vi "2_AdvancedDemo_HHHisto.vi"() -> ()   [LabVIEW 2010]
uses:
  Types/HH_UIThread_Cmds.ctl
  _lib/PQ/HydraHarp/HH_InitInfo.ctl
  Types/HH_UIThread_Data.ctl
  Types/HH_InputChannel.ctl
  _lib/PQ/HydraHarp/HH_RefSource.ctl
  _lib/PQ/HydraHarp/HH_MeasMode.ctl
  _lib/PQ/HydraHarp/hhlib_x86_x64_UIThread.llb/HH_DllPath_global.vi
  <vilib>/Utility/error.llb/DialogType.ctl
  _lib/PQ/HydraHarp/HH_LibVersion_global.vi
panel:
  in  "Settings":bool=TRUE
  in  "Run continuously":bool=TRUE caption="Conti."
  in  "Start":bool
  in  "Scale":bool
  out "CountRates":i32[](graph)
  in  "HistoLength":i32(ring)=6 caption="Num Bins" items=["1024", "2048", "4096", "8192", "16384", "32768", "65536"]
  in  "OvlLevel":u32=4294967295 caption="Ovl.Level" min=1 step=1
  in  "StopOvl.":bool=TRUE
  in  "AcqTime":i32=1000 caption="Acqu.     ms" min=1 max=360000000 step=1
  in  "Binning":i32(ring) caption="Resol.      ps" items=["1", "2", "4", "8", "16", "32", "64", "128", "256", "512", "1024", "2048", "4096", "8192", "16384", "32768", "65536", "131072", "262144", "524288", "1048576", "2097152", "4194304", "8388608", "16777216", "33554432"]
  in  "HistoOffset":i32 caption="Offset      ns" min=0 max=500000 step=1
  out "HistoGraph":T1(graph)={0.0, "Resolution"=0.001, "Histogram"=array8x1024[8192 elements]}
  in  "SyncZeroX":i32=10 caption="ZeroCr.  mV" min=0 max=40 step=1
  in  "SyncDivider":i32(ring)=3 caption="Divider" items=["1", "2", "4", "8", "16"]
  in  "SyncOffset":i32 caption="Offset      ps" min=-99999 max=99999 step=1
  in  "SyncLevel":i32=50 caption="Level      mV" min=0 max=1000 step=1
  in  "Channels":T2[](array[typedef])=[{"Name"="Inp.Chan 1", "Enable"=TRUE, "Offset"=0, "CFDLevel"=50, "ZeroX"=10}, {"Name"="Inp.Chan 2", "Enable"=TRUE, "Offset"=0, "CFDLevel"=50, "ZeroX"=10}, {"Name"="Inp.Chan 3", "Enable"=TRUE, "Offset"=0, "CFDLevel"=50, "ZeroX"=10}, {"Name"="Inp.Chan 4", "Enable"=TRUE, "Offset"=0, "CFDLevel"=50, "ZeroX"=10}, {"Name"="Inp.Chan 5", "Enable"=TRUE, "Offset"=0, "CFDLevel"=50, "ZeroX"=10}, {"Name"="Inp.Chan 6", "Enable"=TRUE, "Offset"=0, "CFDLevel"=50, "ZeroX"=10}, {"Name"="Inp.Chan 7", "Enable"=TRUE, "Offset"=0, "CFDLevel"=50, "ZeroX"=10}, {"Name"="Inp.Chan 8", "Enable"=TRUE, "Offset"=0, "CFDLevel"=50, "ZeroX"=10}] {"ZeroX" min=0 max=40 step=1; "Offset" min=-99999 max=99999 step=1; "CFDLevel" min=0 max=1000 step=1}
  out "SyncRate":string="Sync Rate: 0 cps\n"
  out "OverFlow":bool caption="Overflow:"
  out "Status":string="Initialized!"
  # "Histogram"
  # "Sync"
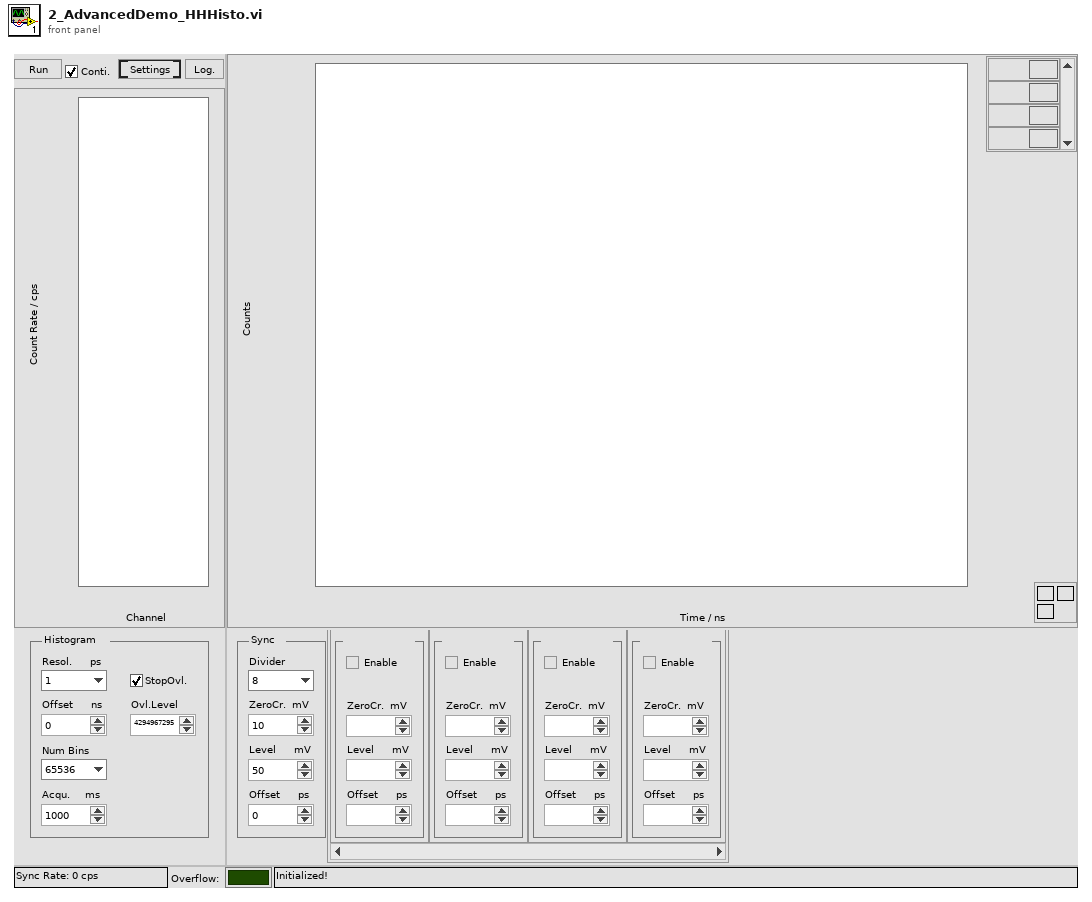
[diagram p1: front panel]
types:
  T1 = cluster{dbl, "Resolution":dbl, "Histogram":u32[][]}
  T2 = typedef "HH_InputChannel.ctl" = cluster{"Name":string, "Enable":bool, "Offset":i32, "CFDLevel":i32, "ZeroX":i32}
  T3 = typedef "HH_UIThread_Data.ctl" = cluster{"Init Info":T4, "DevIdx":i32, "SyncDivider":i32, "SyncOffset":i32, "SyncLevel":i32, "Channels":T2[], "CurrentChannels":i32[], "AcqTime":i32, "Binning":i32, "HistoOffset":i32, "HistoLen":i32, "StopOvl.":bool, "OvlLevel":u32, "StartMeas":bool, "HistoLength":i32, "Resolution":dbl, "Run cont.":bool, "Status":string, "SyncRate":i32, "BitShift":i32, "HistoAcqTime":dbl, "SyncZeroX":i32, "SyncRateStart":i32}
  T4 = typedef "HH_InitInfo.ctl" = cluster{"Library Version":string, "Serial No.":string, "Model":string, "Partnum":string, "Version":string, "features":i32, "nchannels":i32, "nummod":i32, "Model Codes":i32[], "Version Codes":i32[], "Base Resolution":dbl, "Bin Steps":i32}
  T5 = typedef "HH_UIThread_Cmds.ctl" = enum16{"Idle", "Init", "SetInpChanEnable", "SetInpChanOffset", "SetInpChanTrg", "SetSyncDivider", "SetSyncTrg", "SetSyncOffset", "SetBinning", "SetHistoOffset", "SetHistoLen", "SetStopOvl", "SetBitShift", "SetHistoAcqTime", "GetRates", "StartMeas", "StopMeas", "AbortMeas", "GetResolution", "GetHisto", "ReadFiFo", "WriteStatus", "Resize", "EnableControls", "DisableControls", "Error", "Exit"}
  T6 = enum8{"Enabled", "Disabled", "Disabled and Grayed Out"}
  T7 = typedef "HH_MeasMode.ctl" = i32
  T8 = typedef "HH_RefSource.ctl" = enum16{"internal", "external"}
  T9 = typedef "DialogType.ctl" = u16
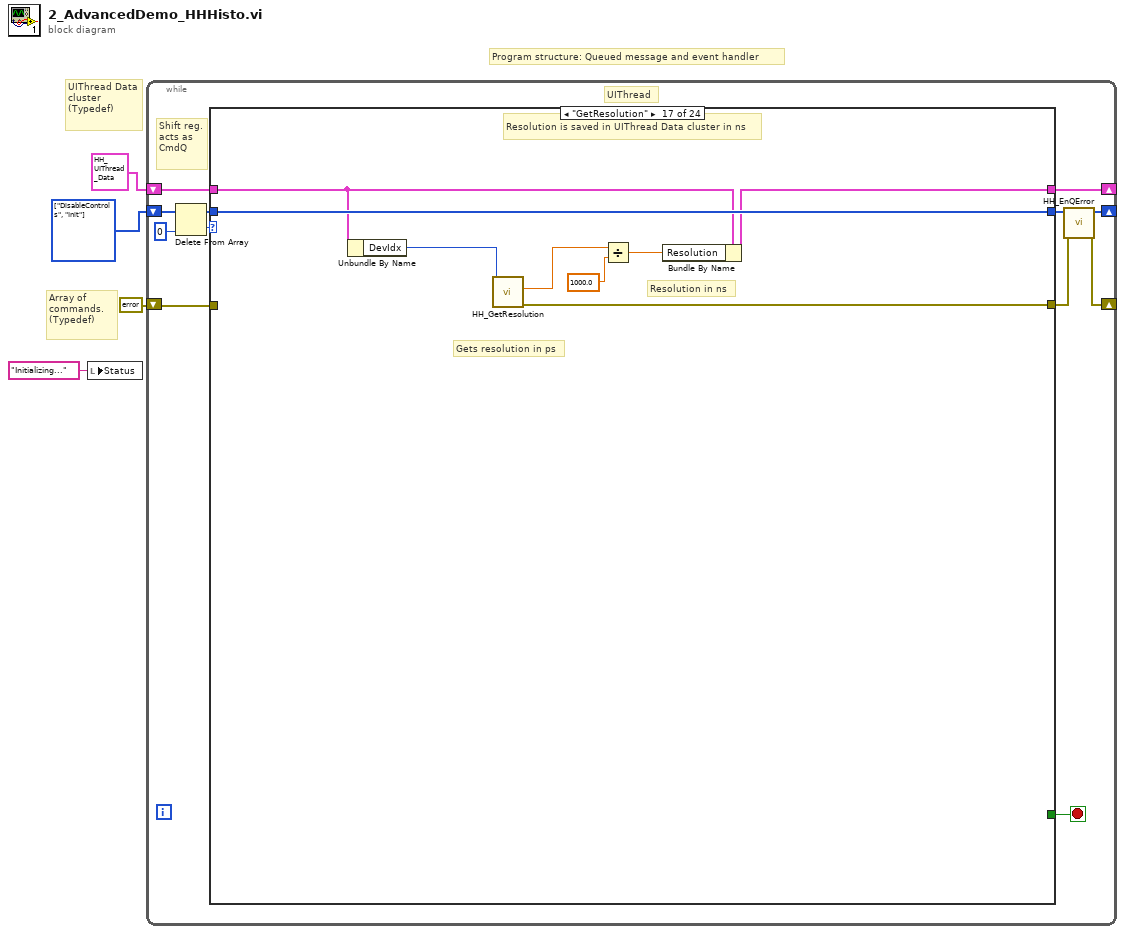
[diagram p0: block diagram]
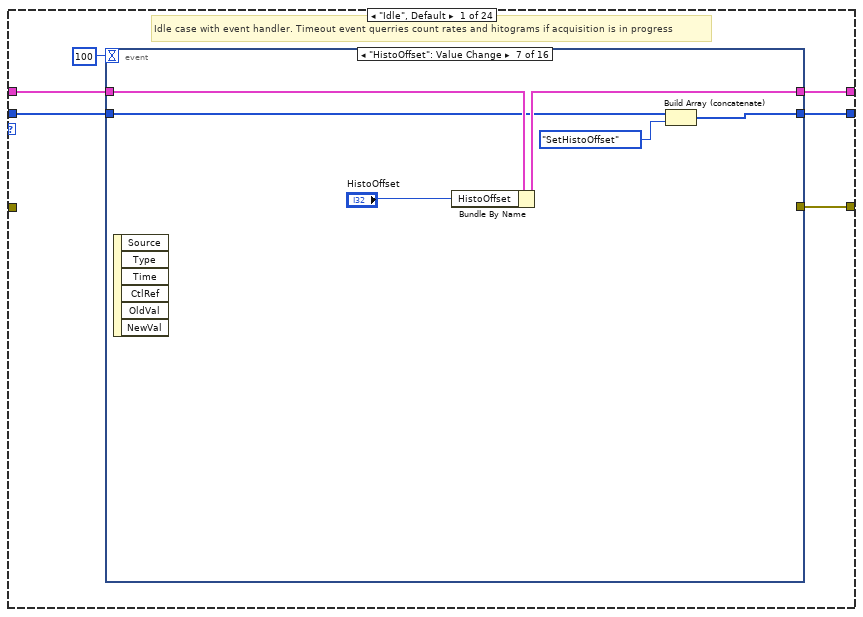
[diagram p2: hidden frame]
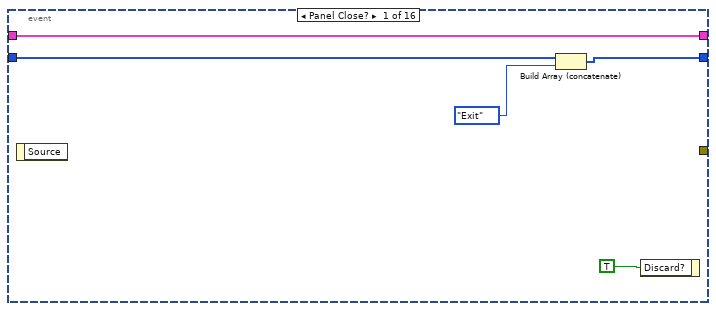
[diagram p3: hidden frame]
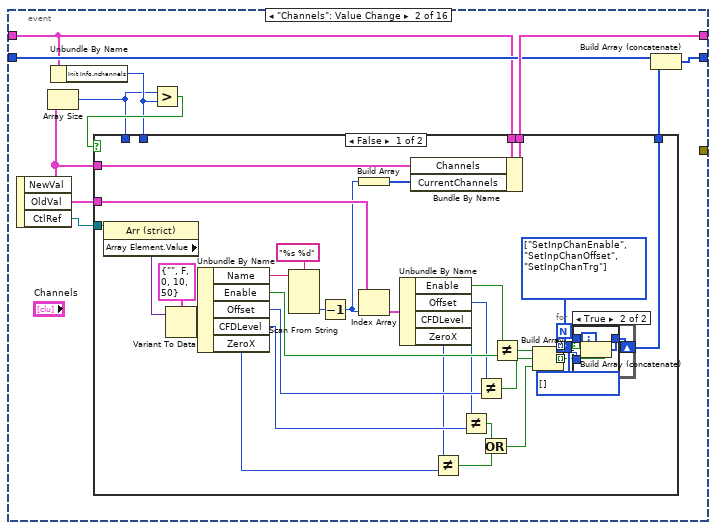
[diagram p4: hidden frame]
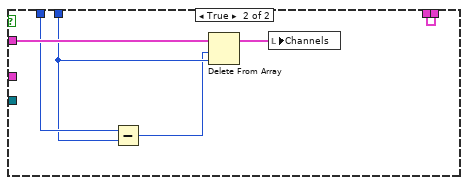
[diagram p6: hidden frame]
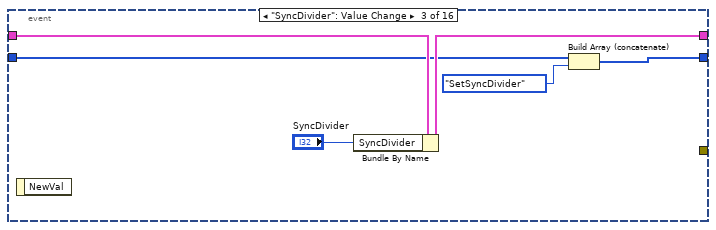
[diagram p7: hidden frame]
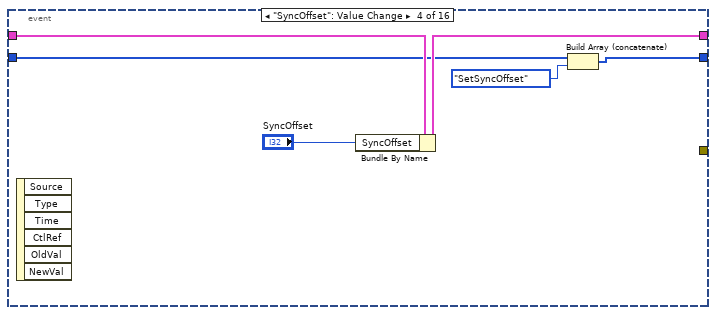
[diagram p8: hidden frame]
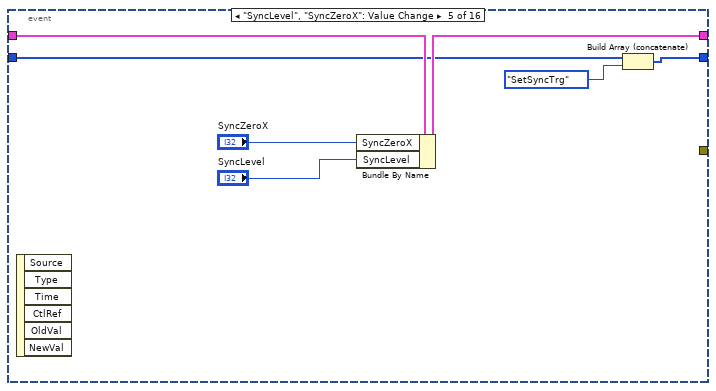
[diagram p9: hidden frame]
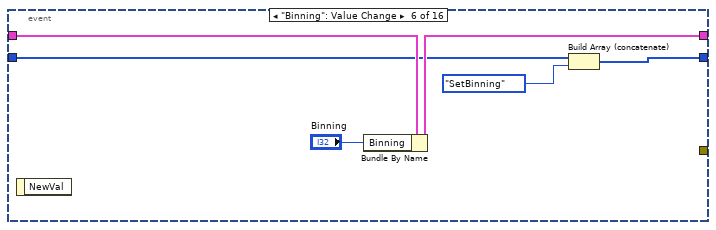
[diagram p10: hidden frame]
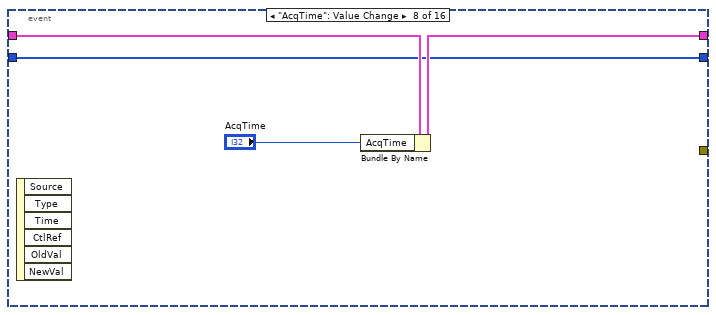
[diagram p11: hidden frame]
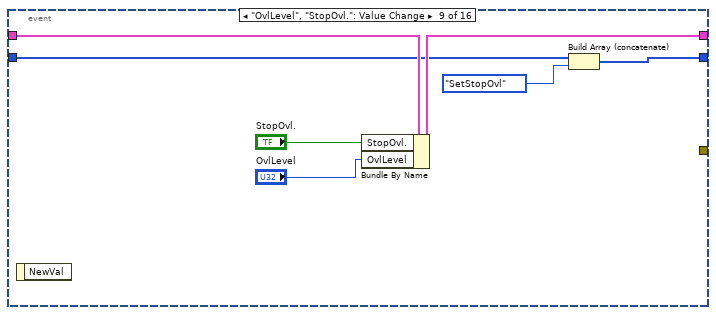
[diagram p12: hidden frame]
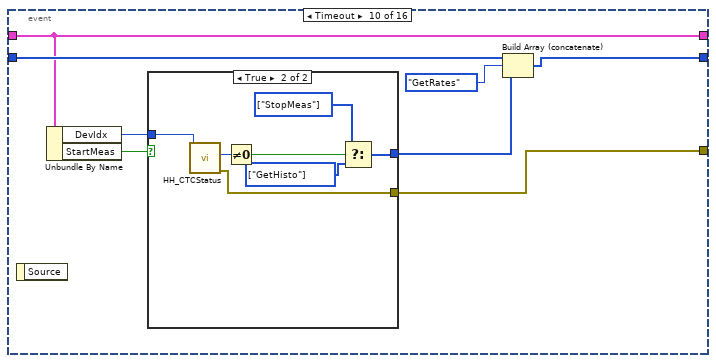
[diagram p13: hidden frame]
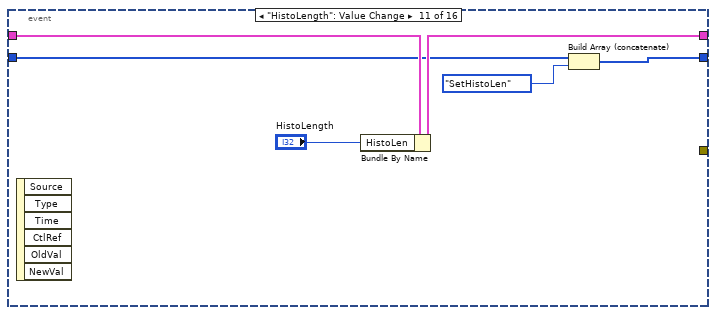
[diagram p15: hidden frame]
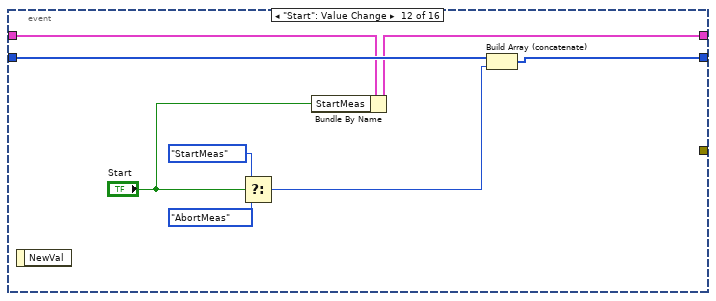
[diagram p16: hidden frame]
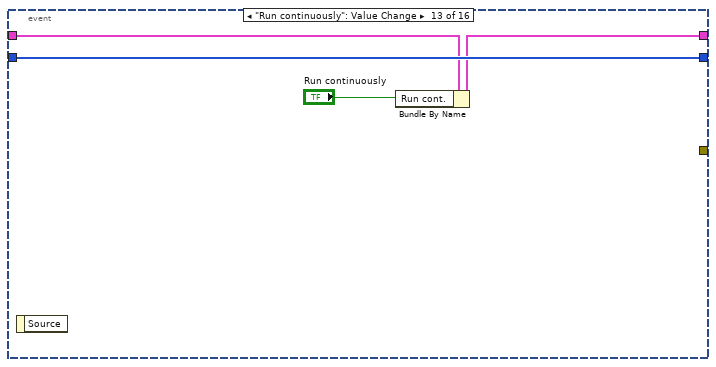
[diagram p17: hidden frame]
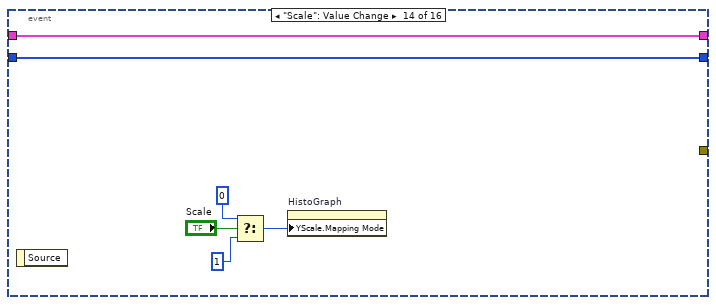
[diagram p18: hidden frame]
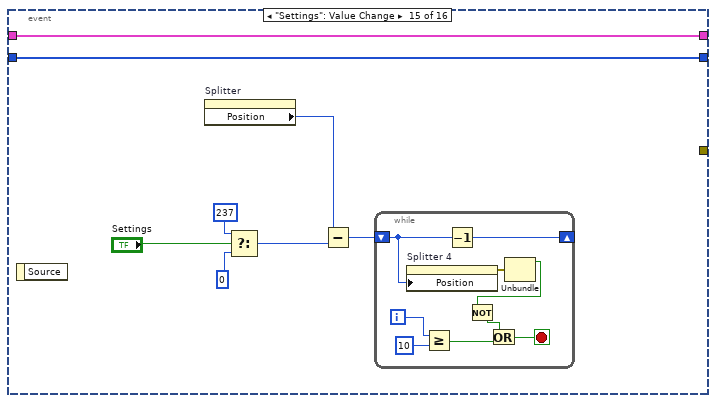
[diagram p19: hidden frame]
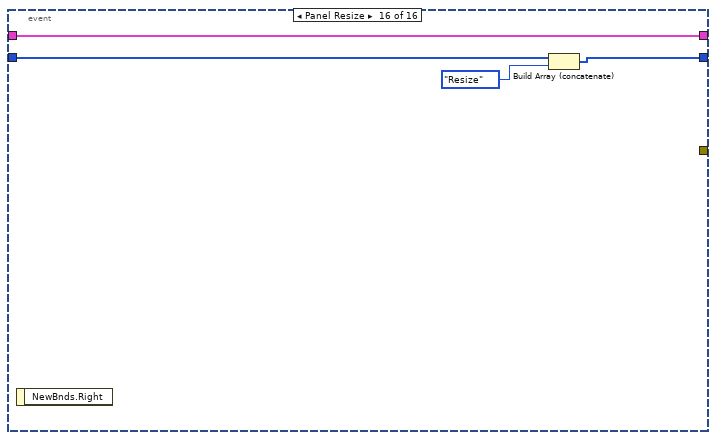
[diagram p20: hidden frame]
diagram:
  w3 = T5[] [enum."DisableControls", enum."Init"] items=["Idle", "Init", "SetInpChanEnable", "SetInpChanOffset", "SetInpChanTrg", "SetSyncDivider", "SetSyncTrg", "SetSyncOffset", "SetBinning", "SetHistoOffset", "SetHistoLen", "SetStopOvl", "SetBitShift", "SetHistoAcqTime", "GetRates", "StartMeas", "StopMeas", "AbortMeas", "GetResolution", "GetHisto", "ReadFiFo", "WriteStatus", "Resize", "EnableControls", "DisableControls", "Error", "Exit"]
  # "Array of commands.\n(Typedef)"
  # "Program structure: Queued message and event handler"
  # "UIThread Data cluster\n(Typedef)"
  n1 = local write "Status"("Initializing..." ("Status")) -> ()
  n2 = while {
    shift-right: [w5] -> _
    shift-left: w3 -> [w12]
    shift-right: [w15] -> _
    shift-left: T3 {"Init Info"={"Library Version"="", "Serial No."="", "Model"="", "Partnum"="", "Version"="", "features"=0, "nchannels"=0, "nummod"=0, "Model Codes"=[], "Version Codes"=[], "Base Resolution"=0.0, "Bin Steps"=0}, "DevIdx"=0, "SyncDivider"=1, "SyncOffset"=0, "SyncLevel"=50, "Channels"=[], "CurrentChannels"=[], "AcqTime"=1, "Binning"=1, "HistoOffset"=1, "HistoLen"=1024, "StopOvl."=FALSE, "OvlLevel"=1024, "StartMeas"=FALSE, "HistoLength"=0, "Resolution"=0.0, "Run cont."=FALSE, "Status"="", "SyncRate"=0, "BitShift"=0, "HistoAcqTime"=0.0, "SyncZeroX"=10, "SyncRateStart"=0} -> [w14]
    shift-right: [w7] -> _
    shift-left: errorcluster {"status"=FALSE, "code"=0, "source"=""} ("error IO") -> [w13]
    stop <- w16 stop-if-true
    # "Shift reg.\nacts as\nCmdQ"
    # "UIThread"
    n3 = Delete From Array(array=w12, index=0) -> (deleted portion=w10:T5, array with subset deleted=w9:T5[])  [unwired: 1 in]
    n4 = case shown="\"GetResolution\"" w10 {
      tunnel: [w22 w232 w255 w269 w283 w300 w309 w311 w318 w326 w334 w339 w351 w366 w374 w388 w402 w427 w452 w465 w472 w484 w490 w494] -> w6
      tunnel: [_ _ _ _ _ _ _ _ _ _ _ _ _ _ _ _ _ _ _ _ _ _ _ TRUE] -> w16
      tunnel: [w21 w212 w258 w272 w286 w302 w310 w315 w322 w327 w329 w340 w350 w372 w377 w391 w398 w426 w451 w453 w471 w483 w491 w497] -> w15
      tunnel: w14 -> [w20 w217 w258 w272 w286 w302 w310 w315 w322 w327 w330 w340 w350 w372 w378 w392 w399 w426 w451 w453 w471 w483 w491 w497]
      tunnel: [w17 w235 w256 w270 w284 w298 w308 w314 w321 w325 w333 w338 w349 w371 w380 w394 w400 w422 _ _ _ _ _ w495] -> w8
      tunnel: w13 -> [_ _ _ _ _ _ _ _ _ _ _ _ _ _ _ _ _ _ _ _ _ _ w492 _]
      tunnel: w9 -> [w19 w234 w255 w269 w283 w300 w309 w311 w317 w326 w334 w339 w351 w367 w375 w389 w402 w427 w452 w465 w472 w484 _ w494]
      frame "Idle", Default {
        # "Idle case with event handler. Timeout event querries count rates and hitograms if acquisition is in progress"
        n5 = event shown="[6] \"HistoOffset\": Value Change" {
          selector: _ -> [_ _ _ _ _ _ _ _ _ _ _ _ _ _ _ _]
          dyn-events: _ -> [_ _ _ _ _ _ _ _ _ _ _ _ _ _ _ _]
          timeout: 100 -> [_ _ _ _ _ _ _ _ _ _ _ _ _ _ _ _]
          tunnel: [w23 w33 w84 w90 w97 w104 w110 w115 w121 w131 w142 w150 w158 w164 w172 w182] -> w22
          tunnel: [w26 w36 w88 w94 w101 w107 w113 w117 w124 w130 w145 w148 w156 w163 w171 w185] -> w21
          tunnel: w20 -> [w26 w32 w89 w95 w102 w108 w114 w118 w125 w130 w146 w149 w157 w163 w171 w185]
          tunnel: w19 -> [w25 w35 w86 w92 w99 w106 w112 w115 w123 w133 w144 w152 w158 w164 w172 w183]
          tunnel: [_ _ _ _ _ _ _ _ _ w126 _ _ _ _ _ _] -> w17
          event Panel Close? {
            n6 = event-data() -> ()  [unwired: 1 in, 1 out]
            n7 = Build Array (concatenate)(w25, HH_UIThread_Cmds."Exit") -> (w23:T5[])
            n8 = event-data("Discard?"=TRUE) -> ()  [unwired: 1 in, 1 out]
          }
          event "Channels": Value Change {
            n9 = event-data() -> ("NewVal"=w31:T2[], "OldVal"=w37:T2[], "CtlRef"=w38:refnum<vi>)  [unwired: 1 in]
            n10 = Array Size(array=w31) -> (size(s)=w28:i32)
            n11 = Unbundle By Name(w32) -> ("Init Info.nchannels"=w29:i32)
            n12 = Greater?(x=w28, y=w29) -> (0:w30:bool)
            n13 = case shown="False" w30 {
              tunnel: w38 -> [w69 _]
              tunnel: w37 -> [w63 _]
              tunnel: [w46 w83] -> w36
              tunnel: [w44 _] -> w34
              tunnel: w32 -> [w41 w83]
              tunnel: w31 -> [w40 w82]
              tunnel: w29 -> [_ w80]
              tunnel: w28 -> [_ w81]
              frame False {
                w39 = T5[] [] items=["Idle", "Init", "SetInpChanEnable", "SetInpChanOffset", "SetInpChanTrg", "SetSyncDivider", "SetSyncTrg", "SetSyncOffset", "SetBinning", "SetHistoOffset", "SetHistoLen", "SetStopOvl", "SetBitShift", "SetHistoAcqTime", "GetRates", "StartMeas", "StopMeas", "AbortMeas", "GetResolution", "GetHisto", "ReadFiFo", "WriteStatus", "Resize", "EnableControls", "DisableControls", "Error", "Exit"] ("Array")
                w47 = T5[] [enum."SetInpChanEnable", enum."SetInpChanOffset", enum."SetInpChanTrg"] items=["Idle", "Init", "SetInpChanEnable", "SetInpChanOffset", "SetInpChanTrg", "SetSyncDivider", "SetSyncTrg", "SetSyncOffset", "SetBinning", "SetHistoOffset", "SetHistoLen", "SetStopOvl", "SetBitShift", "SetHistoAcqTime", "GetRates", "StartMeas", "StopMeas", "AbortMeas", "GetResolution", "GetHisto", "ReadFiFo", "WriteStatus", "Resize", "EnableControls", "DisableControls", "Error", "Exit"]
                n14 = property class="Arr (strict)"(reference=w69) -> ("Array Element.Value"=w68:variant)  [unwired: 1 in, 2 out]
                n15 = Variant To Data(Variant=w68, type=T2 {"Name"="", "Enable"=FALSE, "Offset"=0, "CFDLevel"=10, "ZeroX"=50} ("Channel")) -> (data=w45:cluster{})  [unwired: 1 in, 1 out]
                n16 = Unbundle By Name(w45) -> ("Name"=w66:string, "Enable"=w60:bool, "Offset"=w58:i32, "CFDLevel"=w56:i32, "ZeroX"=w54:i32)
                n17 = Scan From String(format string="%s %d", input string=w66) -> (output 2=w64:i32)  [unwired: 5 in, 3 out]
                n18 = Decrement(x=w64) -> (x-1=w43:i32)
                n19 = Build Array(w43) -> (w42:i32[])
                n20 = Index Array(array=w63, index=w43) -> (element=w62:T2)
                n21 = Unbundle By Name(w62) -> ("Enable"=w61:bool, "Offset"=w59:i32, "CFDLevel"=w57:i32, "ZeroX"=w55:i32)
                n22 = Bundle By Name(cluster=w41, "Channels"=w40, "CurrentChannels"=w42) -> (w46:T3)
                n23 = Not Equal?(x=w55, y=w54) -> (x != y?=w49:bool)
                n24 = Not Equal?(x=w57, y=w56) -> (x != y?=w50:bool)
                n25 = Not Equal?(x=w59, y=w58) -> (x != y?=w52:bool)
                n26 = Or(x=w50, y=w49) -> (x .or. y?=w48:bool)
                n27 = Not Equal?(x=w61, y=w60) -> (x != y?=w53:bool)
                n28 = Build Array(w53, w52, w48) -> (w51:bool[])
                n29 = for {
                  tunnel: w51 -> [w72] mode=indexing
                  tunnel: w47 -> [w73] mode=indexing
                  shift-right: [w70] -> w44
                  shift-left: w39 -> [w71]
                  n30 = case shown="True" w72 {
                    tunnel: w71 -> [w74 w76]
                    tunnel: w73 -> [_ w75]
                    tunnel: [w74 w77] -> w70
                    frame False {
                    }
                    frame True {
                      n31 = Build Array (concatenate)(w76, w75) -> (w77:T5[])
                    }
                  }
                }
              }
              frame True {
                n32 = Subtract(x=w81, y=w80) -> (x-y=w79:i32)
                n33 = Delete From Array(array=w82, length=w79, index=w80) -> (array with subset deleted=w78:T2[])  [unwired: 1 out]
                n34 = local write "Channels"(w78) -> ()
              }
            }
            n35 = Build Array (concatenate)(w35, w34) -> (w33:T5[])
          }
          event "SyncDivider": Value Change {
            n36 = event-data() -> ()  [unwired: 1 in, 1 out]
            n37 = Bundle By Name(cluster=w89, "SyncDivider"="SyncDivider") -> (w88:T3)
            n38 = Build Array (concatenate)(w86, HH_UIThread_Cmds."SetSyncDivider") -> (w84:T5[])
          }
          event "SyncOffset": Value Change {
            n39 = event-data() -> ()  [unwired: 1 in, 6 out]
            n40 = Bundle By Name(cluster=w95, "SyncOffset"="SyncOffset") -> (w94:T3)
            n41 = Build Array (concatenate)(w92, HH_UIThread_Cmds."SetSyncOffset") -> (w90:T5[])
          }
          event "SyncLevel", "SyncZeroX": Value Change {
            n42 = event-data() -> ()  [unwired: 1 in, 6 out]
            n43 = Bundle By Name(cluster=w102, "SyncZeroX"="SyncZeroX", "SyncLevel"="SyncLevel") -> (w101:T3)
            n44 = Build Array (concatenate)(w99, HH_UIThread_Cmds."SetSyncTrg") -> (w97:T5[])
          }
          event "Binning": Value Change {
            n45 = event-data() -> ()  [unwired: 1 in, 1 out]
            n46 = Bundle By Name(cluster=w108, "Binning"="Binning") -> (w107:T3)
            n47 = Build Array (concatenate)(w106, HH_UIThread_Cmds."SetBinning") -> (w104:T5[])
          }
          event "HistoOffset": Value Change {
            n48 = event-data() -> ()  [unwired: 1 in, 6 out]
            n49 = Bundle By Name(cluster=w114, "HistoOffset"="HistoOffset") -> (w113:T3)
            n50 = Build Array (concatenate)(w112, HH_UIThread_Cmds."SetHistoOffset") -> (w110:T5[])
          }
          event "AcqTime": Value Change {
            n51 = event-data() -> ()  [unwired: 1 in, 6 out]
            n52 = Bundle By Name(cluster=w118, "AcqTime"="AcqTime") -> (w117:T3)
          }
          event "OvlLevel", "StopOvl.": Value Change {
            n53 = event-data() -> ()  [unwired: 1 in, 1 out]
            n54 = Bundle By Name(cluster=w125, "StopOvl."="StopOvl.", "OvlLevel"="OvlLevel") -> (w124:T3)
            n55 = Build Array (concatenate)(w123, HH_UIThread_Cmds."SetStopOvl") -> (w121:T5[])
          }
          event Timeout {
            n56 = event-data() -> ()  [unwired: 1 in, 1 out]
            n57 = Unbundle By Name(w130) -> ("DevIdx"=w128:i32, "StartMeas"=w129:bool)
            n58 = case shown="True" w129 {
              tunnel: w128 -> [_ w140]
              tunnel: [_ w138] -> w127
              tunnel: [_ w135] -> w126
              frame False {
              }
              frame True {
                w136 = T5[] [enum."GetHisto"] items=["Idle", "Init", "SetInpChanEnable", "SetInpChanOffset", "SetInpChanTrg", "SetSyncDivider", "SetSyncTrg", "SetSyncOffset", "SetBinning", "SetHistoOffset", "SetHistoLen", "SetStopOvl", "SetBitShift", "SetHistoAcqTime", "GetRates", "StartMeas", "StopMeas", "AbortMeas", "GetResolution", "GetHisto", "ReadFiFo", "WriteStatus", "Resize", "EnableControls", "DisableControls", "Error", "Exit"]
                w137 = T5[] [enum."StopMeas"] items=["Idle", "Init", "SetInpChanEnable", "SetInpChanOffset", "SetInpChanTrg", "SetSyncDivider", "SetSyncTrg", "SetSyncOffset", "SetBinning", "SetHistoOffset", "SetHistoLen", "SetStopOvl", "SetBitShift", "SetHistoAcqTime", "GetRates", "StartMeas", "StopMeas", "AbortMeas", "GetResolution", "GetHisto", "ReadFiFo", "WriteStatus", "Resize", "EnableControls", "DisableControls", "Error", "Exit"]
                n59 = call "HH_CTCStatus.vi"("devidx"=w140) -> ("error out"=w135:errorcluster, "ctcstatus"=w139:i32)  [unwired: 8 in, 1 out]
                n60 = Not Equal To 0?(x=w139) -> (x != 0?=w134:bool)
                n61 = Select(t=w137, s=w134, f=w136) -> (s? t:f=w138:T5[])
              }
            }
            n62 = Build Array (concatenate)(w133, HH_UIThread_Cmds."GetRates", w127) -> (w131:T5[])
          }
          event "HistoLength": Value Change {
            n63 = event-data() -> ()  [unwired: 1 in, 6 out]
            n64 = Bundle By Name(cluster=w146, "HistoLen"="HistoLength") -> (w145:T3)
            n65 = Build Array (concatenate)(w144, HH_UIThread_Cmds."SetHistoLen") -> (w142:T5[])
          }
          event "Start": Value Change {
            n66 = event-data() -> ()  [unwired: 1 in, 1 out]
            n67 = Select(t=HH_UIThread_Cmds."StartMeas", s="Start", f=HH_UIThread_Cmds."AbortMeas") -> (s? t:f=w151:T5)
            n68 = Bundle By Name(cluster=w149, "StartMeas"="Start") -> (w148:T3)
            n69 = Build Array (concatenate)(w152, w151) -> (w150:T5[])
          }
          event "Run continuously": Value Change {
            n70 = event-data() -> ()  [unwired: 1 in, 1 out]
            n71 = Bundle By Name(cluster=w157, "Run cont."="Run continuously") -> (w156:T3)
          }
          event "Scale": Value Change {
            n72 = event-data() -> ()  [unwired: 1 in, 1 out]
            n73 = Select(t=u8 0 ("Y Scale.Mapping Mode"), s="Scale", f=u8 1 ("Y Scale.Mapping Mode")) -> (s? t:f=w159:u8)
            n74 = property on="HistoGraph" class="WFGraph (strict)"("YScale.Mapping Mode"=w159) -> ()  [unwired: 2 in, 2 out]
          }
          event "Settings": Value Change {
            n75 = event-data() -> ()  [unwired: 1 in, 1 out]
            n76 = property on="Splitter" class="Splitter"() -> ("Position"=w170:i32)  [unwired: 2 in, 2 out]
            n77 = Select(t=237 ("PosT"), s="Settings", f=0 ("PosF")) -> (s? t:f=w167:i32)
            n78 = Subtract(x=w170, y=w167) -> (x-y=w166:i32)
            n79 = while {
              shift-right: [w181] -> _
              shift-left: w166 -> [w174]
              i -> [w180]
              stop <- w177 stop-if-true
              n80 = property on="Splitter 4" class="Splitter"("Position"=w174) -> (error out=w173:errorcluster)  [unwired: 2 in, 1 out]
              n81 = Greater Or Equal?(x=w180, y=10) -> (x >= y?=w178:bool)
              n82 = Decrement(x=w174) -> (x-1=w181:i32)
              n83 = Unbundle(w173) -> ("status"=w176:bool)  [unwired: 2 out]
              n84 = Not(x=w176) -> (.not. x?=w175:bool)
              n85 = Or(x=w175, y=w178) -> (x .or. y?=w177:bool)
            }
          }
          event Panel Resize {
            n86 = event-data() -> ()  [unwired: 1 in, 1 out]
            n87 = Build Array (concatenate)(w183, HH_UIThread_Cmds."Resize") -> (w182:T5[])
          }
        }
      }
      frame "Init" {
        w204 = T7 0 items=["Histo"=0, "T2"=2, "T3"=3, "Conti"=8]  # mode
        w203 = HH_RefSource."internal"  # refsource
        w219 = TRUE ("Run cont.")
        w221 = FALSE ("StartMeas")
        w222 = u32 100000 ("OvlLevel")
        w223 = TRUE ("StopOvl.")
        w224 = 6 ("HistoLen")
        w225 = 1000 ("AcqTime")
        w226 = 0 ("HistoOffset")
        w227 = 0 ("Binning")
        w228 = 50 ("SyncLevel")
        w229 = 10 ("SyncZeroX")
        w230 = 0 ("SyncOffset")
        w231 = 3 ("SyncDivider")
        w233 = T5[] [enum."SetSyncDivider", enum."SetSyncOffset", enum."SetSyncTrg", enum."SetInpChanEnable", enum."SetInpChanOffset", enum."SetInpChanTrg", enum."SetBinning", enum."SetHistoOffset", enum."SetHistoLen", enum."SetStopOvl", enum."Resize", enum."EnableControls", enum."WriteStatus"] items=["Idle", "Init", "SetInpChanEnable", "SetInpChanOffset", "SetInpChanTrg", "SetSyncDivider", "SetSyncTrg", "SetSyncOffset", "SetBinning", "SetHistoOffset", "SetHistoLen", "SetStopOvl", "SetBitShift", "SetHistoAcqTime", "GetRates", "StartMeas", "StopMeas", "AbortMeas", "GetResolution", "GetHisto", "ReadFiFo", "WriteStatus", "Resize", "EnableControls", "DisableControls", "Error", "Exit"]
        # "Init HW"
        # "Set path to mhlib.dll"
        # "Init all FP controls and corresponding copy in UIThread Data cluster"
        # "EnQ list of commands"
        # "Array with Inp.Chan."
        # "Initialization: 1. Init HW -> get # of channels -> make array for Inp.Channels\n2. Init all FP controls and corresponding fields in UIThread Data cluster\n3. EnQ list of commands for further initialization"
        n88 = call <vilib>:"Error Cluster From Error Code.vi"("is warning? (False)"=FALSE, "show call chain? (False)"=TRUE, "error message (\"\")"="DLL not found!" ("error message (\"\")"), "error code (0)"=5000) -> ("error out"=w205:errorcluster)  [unwired: 5 in]
        n89 = call "GetDLLPath.vi"("DllName_32bit"="HHLib.dll" ("name or relative path"), "DllName_64bit"="HHLib64.dll" ("name or relative path")) -> ("file exists?"=w207:bool, "DLLPath"=w208:path)  [unwired: 8 in]
        n90 = global write "HH_DllPath_global.vi" "DllPath"(w208) -> ()
        n91 = Build Array (concatenate)(w234, w233) -> (w232:T5[])
        n92 = Select(t=errorcluster {"status"=FALSE, "code"=0, "source"=""} ("error IO"), s=w207, f=w205) -> (s? t:f=w213:errorcluster)
        n93 = global read "HH_LibVersion_global.vi" "Library Version"() -> (w202:string)
        n94 = call "InitHH_UIThread.vi"("error in (no error)"=w213, "mode"=w204, "refsource"=w203, "Library Version"=w202) -> ("error out"=w235:errorcluster, "Init Info"=w238:T4, "DevIdx"=w237:i32)  [unwired: 5 in]
        n95 = local write "SyncDivider"(w231) -> ()
        n96 = local write "SyncOffset"(w230) -> ()
        n97 = local write "SyncZeroX"(w229) -> ()
        n98 = local write "SyncLevel"(w228) -> ()
        n99 = local write "Binning"(w227) -> ()
        n100 = local write "HistoOffset"(w226) -> ()
        n101 = local write "HistoLength"(w224) -> ()
        n102 = local write "StopOvl."(w223) -> ()
        n103 = local write "OvlLevel"(w222) -> ()
        n104 = local write "Start"(w221) -> ()
        n105 = local write "Run continuously"(w219) -> ()
        n106 = local write "AcqTime"(w225) -> ()
        n107 = Bundle By Name(cluster=w217, "DevIdx"=w237, "Init Info"=w238, "Status"="Initialized!") -> (w216:T3)
        n108 = Unbundle By Name(w216) -> ("Init Info.Bin Steps"=w215:i32, "Init Info.nchannels"=w191:i32, "Init Info.Base Resolution"=w196:dbl)
        n109 = Initialize Array(u32 0, w191, 1024 ("dimension size")) -> (w195:u32[][])
        n110 = Divide(x=w196, y=1000.0) -> (x/y=w197:dbl)
        n111 = call "HH_CalcBinningValues.vi"("Bin Steps"=w215) -> ("BinningValues"=w220:cluster{"String":string, "Value":i32}[])  [unwired: 10 in]
        n112 = property on="Binning" class="Ring (strict)"("StringsAndValues[]"=w220) -> ()  [unwired: 2 in, 2 out]
        n113 = Bundle(0.0, w197, w195) -> (w194:cluster{dbl, dbl, u32[][]})  [unwired: 1 in]
        n114 = for {
          N: w191 -> [_]
          tunnel: T2 {"Name"="", "Enable"=FALSE, "Offset"=0, "CFDLevel"=10, "ZeroX"=50} ("Channel") -> [w251]
          tunnel: [w250] -> w190 mode=indexing
          tunnel: [w240] -> w192 mode=indexing
          tunnel: w194 -> [w241]
          i -> [w240]
          # "Init values for Inp. Channels"
          n115 = Increment(x=w240) -> (x+1=w239:i32)
          n116 = Format Into String(format string="Inp.Chan %d", w239) -> (resulting string=w248:string)  [unwired: 2 in, 1 out]
          n117 = Format Into String(format string="Ch.%d", w239) -> (resulting string=w242:string)  [unwired: 2 in, 1 out]
          n118 = Bundle By Name(cluster=w251, "Name"=w248, "Enable"=TRUE, "Offset"=0, "CFDLevel"=50 ("CFDZeroX"), "ZeroX"=10 ("CFDLevel")) -> (w250:T2)
          n119 = property on="HistoGraph" class="WFGraph (strict)"("Value"=w241, "Active Plot"=w240, "Plot.Plot Name"=w242) -> ()  [unwired: 2 in, 2 out]
        }
        n120 = local write "Channels"(w190) -> ()
        n121 = Bundle By Name(cluster=w216, "Channels"=w190, "CurrentChannels"=w192, "SyncDivider"=w231, "SyncOffset"=w230, "SyncZeroX"=w229, "SyncLevel"=w228, "Binning"=w227, "HistoOffset"=w226, "AcqTime"=w225, "HistoLen"=w224, "StopOvl."=w223, "OvlLevel"=w222, "StartMeas"=w221, "Run cont."=w219) -> (w212:T3)
        n122 = property on="HistoGraph" class="WFGraph (strict)"("LegPlotMin"=u32 4 ("Legend:Plot Minimum")) -> ()  [unwired: 2 in, 2 out]
        n123 = property on="Settings" class="Bool (strict)"("Val(Sgnl)"=TRUE ("Value (Signaling)")) -> ()  [unwired: 2 in, 2 out]
        n124 = property on="Scale" class="Bool (strict)"("Val(Sgnl)"=FALSE ("Value (Signaling)")) -> ()  [unwired: 2 in, 2 out]
      }
      frame "SetInpChanEnable" {
        n125 = Unbundle By Name(w258) -> ("DevIdx"=w257:i32, "Channels"=w252:T2[], "CurrentChannels"=w253:i32[])
        n126 = for {
          tunnel: w257 -> [w265]
          shift-right: [w264] -> w256
          shift-left: errorcluster {"status"=FALSE, "code"=0, "source"=""} ("error out") -> [w263]
          tunnel: w253 -> [w259] mode=indexing
          tunnel: w252 -> [w262]
          n127 = Index Array(array=w262, index=w259) -> (element=w261:T2)
          n128 = Unbundle By Name(w261) -> ("Enable"=w260:bool)
          n129 = call "HH_SetInputChannelEnable.vi"("error in (no error)"=w263, "enable"=w260, "channel"=w259, "devidx"=w265) -> ("error out"=w264:errorcluster)  [unwired: 6 in, 1 out]
        }
      }
      frame "SetInpChanOffset" {
        n130 = Unbundle By Name(w272) -> ("DevIdx"=w271:i32, "Channels"=w266:T2[], "CurrentChannels"=w267:i32[])
        n131 = for {
          tunnel: w271 -> [w277]
          shift-right: [w274] -> w270
          shift-left: errorcluster {"status"=FALSE, "code"=0, "source"=""} ("error out") -> [w275]
          tunnel: w267 -> [w276] mode=indexing
          tunnel: w266 -> [w279]
          n132 = Index Array(array=w279, index=w276) -> (element=w278:T2)
          n133 = Unbundle By Name(w278) -> ("Offset"=w273:i32)
          n134 = call "HH_SetInputChannelOffset.vi"("error in (no error)"=w275, "Offset"=w273, "channel"=w276, "devidx"=w277) -> ("error out"=w274:errorcluster)  [unwired: 6 in, 1 out]
        }
      }
      frame "SetInpChanTrg" {
        n135 = Unbundle By Name(w286) -> ("DevIdx"=w285:i32, "Channels"=w280:T2[], "CurrentChannels"=w281:i32[])
        n136 = for {
          tunnel: w285 -> [w289]
          shift-right: [w291] -> w284
          shift-left: errorcluster {"status"=FALSE, "code"=0, "source"=""} ("error out") -> [w292]
          tunnel: w281 -> [w290] mode=indexing
          tunnel: w280 -> [w294]
          n137 = Index Array(array=w294, index=w290) -> (element=w293:T2)
          n138 = Unbundle By Name(w293) -> ("CFDLevel"=w288:i32, "ZeroX"=w287:i32)
          n139 = call "HH_SetInputCFD.vi"("CFD Channel"=w290, "error in (no error)"=w292, "CFD ZeroCross"=w287, "CFD Level"=w288, "devidx"=w289) -> ("error out"=w291:errorcluster)  [unwired: 5 in, 1 out]
        }
      }
      frame "SetSyncDivider" {
        n140 = Unbundle By Name(w302) -> ("DevIdx"=w301:i32, "SyncDivider"=w297:i32)
        n141 = Power Of 2(x=w297) -> (2^x=w296:dbl)
        n142 = To Long Integer(number=w296) -> (32bit integer=w295:i32)
        n143 = call "HH_SetSyncDiv.vi"("SyncDivider"=w295, "devidx"=w301) -> ("error out"=w299:errorcluster)  [unwired: 8 in, 1 out]
        n144 = flat-sequence {
          tunnel: w299 -> [w303]
          tunnel: [w303] -> w298
          frame #0 {
            n145 = Wait (ms)(milliseconds to wait=u32 100) -> ()  [unwired: 1 out]
          }
        }
      }
      frame "SetSyncTrg" {
        n146 = Unbundle By Name(w310) -> ("DevIdx"=w307:i32, "SyncLevel"=w305:i32, "SyncZeroX"=w306:i32)
        n147 = call "HH_SetSyncCFD.vi"("CFD ZeroCross"=w306, "CFD Level"=w305, "devidx"=w307) -> ("error out"=w308:errorcluster)  [unwired: 7 in, 1 out]
      }
      frame "SetSyncOffset" {
        n148 = Unbundle By Name(w315) -> ("DevIdx"=w313:i32, "SyncOffset"=w312:i32)
        n149 = call "HH_SetSyncChannelOffset.vi"("Offset"=w312, "devidx"=w313) -> ("error out"=w314:errorcluster)  [unwired: 8 in, 1 out]
      }
      frame "SetBinning" {
        # "When binning is changed the new resolution is querried"
        n150 = Unbundle By Name(w322) -> ("DevIdx"=w320:i32, "Binning"=w319:i32)
        n151 = call "HH_SetBinning.vi"("Binning"=w319, "devidx"=w320) -> ("error out"=w321:errorcluster)  [unwired: 8 in, 1 out]
        n152 = Build Array (concatenate)(HH_UIThread_Cmds."GetResolution", w317) -> (w318:T5[])
      }
      frame "SetHistoOffset" {
        n153 = Unbundle By Name(w327) -> ("DevIdx"=w324:i32, "HistoOffset"=w323:i32)
        n154 = call "HH_SetOffset.vi"("Offset"=w323, "devidx"=w324) -> ("error out"=w325:errorcluster)  [unwired: 8 in, 1 out]
      }
      frame "SetHistoLen" {
        n155 = Unbundle By Name(w330) -> ("DevIdx"=w332:i32, "HistoLen"=w331:i32)
        n156 = call "HH_SetHistoLen.vi"("lencode"=w331, "devidx"=w332) -> ("error out"=w333:errorcluster, "actuallen"=w328:i32)  [unwired: 7 in, 1 out]
        n157 = Bundle By Name(cluster=w330, "HistoLength"=w328) -> (w329:T3)
      }
      frame "SetStopOvl" {
        n158 = Unbundle By Name(w340) -> ("DevIdx"=w337:i32, "StopOvl."=w336:bool, "OvlLevel"=w335:u32)
        n159 = call "HH_SetStopOverflow.vi"("stopcount"=w335, "StopOnOverflow"=w336, "devidx"=w337) -> ("error out"=w338:errorcluster)  [unwired: 7 in, 1 out]
      }
      frame "GetRates" {
        n160 = Unbundle By Name(w350) -> ("Init Info.nchannels"=w348:i32, "Channels"=w341:T2[], "DevIdx"=w342:i32)
        n161 = call "HH_GetSyncRate.vi"("devidx"=w342) -> ("error out"=w347:errorcluster, "syncrate"=w346:i32)  [unwired: 8 in, 1 out]
        n162 = Format Into String(format string="Sync Rate: %d cps\n", w346) -> (resulting string=→"SyncRate":string)  [unwired: 2 in, 1 out]
        n163 = for {
          N: w348 -> [_]
          tunnel: w342 -> [w357]
          tunnel: [w354] -> w344 mode=indexing
          shift-right: [w356] -> w349
          shift-left: w347 -> [w358]
          tunnel: w341 -> [w353] mode=indexing
          i -> [w355]
          n164 = Unbundle By Name(w353) -> ("Enable"=w352:bool)
          n165 = case shown="False" w352 {
            tunnel: w358 -> [w359 w364]
            tunnel: w357 -> [_ w363]
            tunnel: [w359 w362] -> w356
            tunnel: w355 -> [_ w361]
            tunnel: [_ w360] -> w354
            frame False {
            }
            frame True {
              n166 = call "HH_GetCountRate.vi"("error in (no error)"=w364, "Channel"=w361, "devidx"=w363) -> ("error out"=w362:errorcluster, "rate"=w360:i32)  [unwired: 6 in, 1 out]
            }
          }
        }
        "CountRates" <- w344
      }
      frame "StartMeas" {
        n167 = Unbundle By Name(w372) -> ("AcqTime"=w368:i32, "DevIdx"=w369:i32)
        n168 = call "HH_ClearHistMem.vi"("devidx"=w369) -> ("error out"=w370:errorcluster)  [unwired: 9 in, 1 out]
        n169 = call "HH_StartMeas.vi"("error in (no error)"=w370, "tacq"=w368, "devidx"=w369) -> ("error out"=w371:errorcluster)  [unwired: 7 in, 1 out]
        n170 = Build Array (concatenate)(w367, HH_UIThread_Cmds."GetHisto") -> (w366:T5[])
      }
      frame "StopMeas" {
        n171 = Unbundle By Name(w378) -> ("Run cont."=w373:bool, "DevIdx"=w379:i32)
        n172 = call "HH_StopMeas.vi"("devidx"=w379) -> ("error out"=w380:errorcluster)  [unwired: 9 in, 1 out]
        n173 = case shown="True" w373 {
          tunnel: w378 -> [w384 w386]
          tunnel: [w383 w386] -> w377
          tunnel: [w381 w385] -> w376
          frame False {
            w381 = T5[] [enum."GetHisto"] items=["Idle", "Init", "SetInpChanEnable", "SetInpChanOffset", "SetInpChanTrg", "SetSyncDivider", "SetSyncTrg", "SetSyncOffset", "SetBinning", "SetHistoOffset", "SetHistoLen", "SetStopOvl", "SetBitShift", "SetHistoAcqTime", "GetRates", "StartMeas", "StopMeas", "AbortMeas", "GetResolution", "GetHisto", "ReadFiFo", "WriteStatus", "Resize", "EnableControls", "DisableControls", "Error", "Exit"]
            w382 = FALSE ("StartMeas")
            n174 = Bundle By Name(cluster=w384, "StartMeas"=w382) -> (w383:T3)
            n175 = local write "Start"(w382) -> ()
          }
          frame True {
            w385 = T5[] [enum."GetHisto", enum."StartMeas"] items=["Idle", "Init", "SetInpChanEnable", "SetInpChanOffset", "SetInpChanTrg", "SetSyncDivider", "SetSyncTrg", "SetSyncOffset", "SetBinning", "SetHistoOffset", "SetHistoLen", "SetStopOvl", "SetBitShift", "SetHistoAcqTime", "GetRates", "StartMeas", "StopMeas", "AbortMeas", "GetResolution", "GetHisto", "ReadFiFo", "WriteStatus", "Resize", "EnableControls", "DisableControls", "Error", "Exit"]
          }
        }
        n176 = Build Array (concatenate)(w375, w376) -> (w374:T5[])
      }
      frame "AbortMeas" {
        w390 = T5[] [enum."GetHisto"] items=["Idle", "Init", "SetInpChanEnable", "SetInpChanOffset", "SetInpChanTrg", "SetSyncDivider", "SetSyncTrg", "SetSyncOffset", "SetBinning", "SetHistoOffset", "SetHistoLen", "SetStopOvl", "SetBitShift", "SetHistoAcqTime", "GetRates", "StartMeas", "StopMeas", "AbortMeas", "GetResolution", "GetHisto", "ReadFiFo", "WriteStatus", "Resize", "EnableControls", "DisableControls", "Error", "Exit"]
        w387 = FALSE ("StartMeas")
        n177 = Unbundle By Name(w392) -> ("DevIdx"=w393:i32)
        n178 = call "HH_StopMeas.vi"("devidx"=w393) -> ("error out"=w394:errorcluster)  [unwired: 9 in, 1 out]
        n179 = Bundle By Name(cluster=w392, "StartMeas"=w387) -> (w391:T3)
        n180 = local write "Start"(w387) -> ()
        n181 = Build Array (concatenate)(w389, w390) -> (w388:T5[])
      }
      frame "GetResolution" {
        # "Resolution in ns"
        # "Gets resolution in ps"
        # "Resolution is saved in UIThread Data cluster in ns"
        n182 = Unbundle By Name(w399) -> ("DevIdx"=w401:i32)
        n183 = call "HH_GetResolution.vi"("devidx"=w401) -> ("error out"=w400:errorcluster, "resolution"=w397:dbl)  [unwired: 8 in, 1 out]
        n184 = Divide(x=w397, y=1000.0) -> (x/y=w395:dbl)
        n185 = Bundle By Name(cluster=w399, "Resolution"=w395) -> (w398:T3)
      }
      frame "GetHisto" {
        w411 = 1  # FLAG_OVERFLOW
        # "Provides a buffer (U32-array of length 'HistoLength') for histograms."
        n186 = Unbundle By Name(w426) -> ("Resolution"=w423:dbl, "Init Info.nchannels"=w403:i32, "Channels"=w404:T2[], "DevIdx"=w425:i32, "HistoLength"=w424:i32)
        n187 = call "HH_AllocateHistoBuffer.vi"("HistoLength"=w424) -> ("Buffer"=w417:u32[])  [unwired: 10 in]
        n188 = for {
          N: w403 -> [_]
          tunnel: w425 -> [w440]
          tunnel: [w437] -> w414 mode=indexing
          tunnel: w417 -> [w438]
          shift-right: [w439] -> w413
          shift-left: errorcluster {"status"=FALSE, "code"=0, "source"=""} ("error IO") -> [w431]
          shift-right: [w432] -> w406
          shift-left: "Total Counts:\t\t" -> [w430]
          tunnel: w404 -> [w429] mode=indexing
          i -> [w436]
          n189 = Unbundle By Name(w429) -> ("Enable"=w428:bool)
          n190 = case shown="True" w428 {
            tunnel: w440 -> [_ w449]
            tunnel: [w441 w448] -> w439
            tunnel: w438 -> [w442 w446]
            tunnel: [w442 w445] -> w437
            tunnel: w436 -> [_ w444]
            tunnel: w431 -> [w441 w443]
            frame False {
            }
            frame True {
              n191 = call "HH_GetHistogram.vi"("Chcount"=w446, "error in (no error)"=w443, "clear"=0, "channel"=w444, "devidx"=w449) -> ("error out"=w448:errorcluster, "Histogram"=w445:u32[])  [unwired: 4 in, 1 out]
            }
          }
          n192 = Add Array Elements(numeric array=w437) -> (sum=w433:u32)
          n193 = Increment(x=w436) -> (x+1=w434:i32)
          n194 = Format Into String(format string="Ch.%2d: %d cnts.\t\t", initial string=w430, w434, w433) -> (resulting string=w432:string)  [unwired: 1 in, 1 out]
        }
        n195 = call "CalcRate.vi"("Refresh(ms)"=u32 500) -> ("Rate / Hz"=w421:dbl)  [unwired: 8 in, 2 out]
        n196 = Format Into String(format string="Readout Rate: %.1f Hz\\t\\t", w421) -> (resulting string=w419:string)  [unwired: 2 in, 1 out]
        n197 = Concatenate Strings(w419, w406) -> (w418:string)
        n198 = Bundle(0.0, "Resolution"=w423, "Histogram"=w414) -> (→"HistoGraph":T1)  [unwired: 1 in]
        n199 = local write "Status"(w418) -> ()
        n200 = call "HH_GetFlags.vi"("error in (no error)"=w413) -> ("error out"=w422:errorcluster, "flags"=w410:i32)  [unwired: 8 in, 1 out]
        n201 = And(x=w411, y=w410) -> (x .and. y?=w412:i32)
        n202 = Not Equal To 0?(x=w412) -> (x != 0?=→"OverFlow":bool)
      }
      frame "WriteStatus" {
        n203 = Unbundle By Name(w451) -> ("Status"=→"Status":string)
      }
      frame "Resize" {
        n204 = property on="Pane 3" class="Pane"() -> ("Width"=w458:u32)  [unwired: 2 in, 2 out]
        n205 = Subtract(x=w458, y=i16 100 ("b")) -> (x-y=w464:u32)
        n206 = Unbundle By Name(w453) -> ("Init Info.nchannels"=w461:i32)
        n207 = Quotient & Remainder(x=w464, y=i16 99 ("m")) -> (floor(x/y)=w463:u32)  [unwired: 1 out]
        n208 = In Range and Coerce(upper limit=w461, x=w463, lower limit=4) -> (coerced(x)=w462:u32)  [unwired: 1 out]
        n209 = Equal?(x=w461, y=w462) -> (x = y?=w460:bool)
        n210 = Not(x=w460) -> (.not. x?=w459:bool)
        n211 = property on="Channels" class="Arr (strict)"("HorizScroll"=w459, "Number of Columns"=w462, "Index Values"=u32[] [0]) -> ()  [unwired: 2 in, 2 out]
      }
      frame "EnableControls" {
        n212 = property class="VI"() -> ("Panel"=w469:refnum<vi>)  [unwired: 2 in, 2 out]
        n213 = property class="Pnl"(reference=w469) -> ("Controls[]"=w468:refnum<vi>[])  [unwired: 1 in, 2 out]
        n214 = property class="Pnl"(reference=w469) -> ("Decos[]"=w470:refnum<vi>[])  [unwired: 1 in, 2 out]
        n215 = for {
          tunnel: w470 -> [w474] mode=indexing
          tunnel: TRUE -> [w473]
          n216 = property class="Decor"(reference=w474, "Visible"=w473) -> ()  [unwired: 1 in, 2 out]
        }
        n217 = for {
          tunnel: w468 -> [w477] mode=indexing
          tunnel: T6."Enabled" ("Disabled") -> [w476]
          tunnel: [w475] -> _
          n218 = property class="Ctl"(reference=w477, "DisabledEnum"=w476) -> (error out=w475:errorcluster)  [unwired: 1 in, 1 out]
        }
      }
      frame "DisableControls" {
        n219 = property class="VI"() -> ("Panel"=w481:refnum<vi>)  [unwired: 2 in, 2 out]
        n220 = property class="Pnl"(reference=w481) -> ("Controls[]"=w480:refnum<vi>[])  [unwired: 1 in, 2 out]
        n221 = property class="Pnl"(reference=w481) -> ("Decos[]"=w482:refnum<vi>[])  [unwired: 1 in, 2 out]
        n222 = for {
          tunnel: w482 -> [w486] mode=indexing
          tunnel: FALSE -> [w485]
          n223 = property class="Decor"(reference=w486, "Visible"=w485) -> ()  [unwired: 1 in, 2 out]
        }
        n224 = for {
          tunnel: w480 -> [w489] mode=indexing
          tunnel: T6."Disabled and Grayed Out" ("Disabled") -> [w488]
          tunnel: [w487] -> _
          n225 = property class="Ctl"(reference=w489, "DisabledEnum"=w488) -> (error out=w487:errorcluster)  [unwired: 1 in, 1 out]
        }
      }
      frame "Error" {
        w490 = T5[] [enum."Exit"] items=["Idle", "Init", "SetInpChanEnable", "SetInpChanOffset", "SetInpChanTrg", "SetSyncDivider", "SetSyncTrg", "SetSyncOffset", "SetBinning", "SetHistoOffset", "SetHistoLen", "SetStopOvl", "SetBitShift", "SetHistoAcqTime", "GetRates", "StartMeas", "StopMeas", "AbortMeas", "GetResolution", "GetHisto", "ReadFiFo", "WriteStatus", "Resize", "EnableControls", "DisableControls", "Error", "Exit"]
        w493 = T9 1 items=["no dialog", "OK message", "continue or stop message", "OK message + warnings", "continue/stop + warnings"] ("type of dialog (OK msg:1)")
        # "Error case: If an error occures the user is informed and the programm terminates. Add your own code to handle error events (e.g. exception lists, etc.)"
        n226 = call <vilib>:"Simple Error Handler.vi"("type of dialog (OK msg:1)"=w493, "error in (no error)"=w492) -> ()  [unwired: 3 in, 5 out]
      }
      frame "Exit" {
        n227 = Unbundle By Name(w497) -> ("DevIdx"=w496:i32)
        n228 = call "HH_CloseDevice.vi"("devidx"=w496) -> ("error out"=w495:errorcluster)  [unwired: 9 in, 1 out]
      }
    }
    n229 = call "HH_EnQError.vi"("error in (no error)"=w8, "Cmds_in"=w6) -> ("error out"=w7:errorcluster, "Cmds_out"=w5:T5[])  [unwired: 8 in]
  }
